vi "Sift Flush Loop.vi"(8 "error in (no error)":errorcluster, 10 "Stop Notifier":refnum<notifier>, 11 "Sift Client In":refnum<class "Sift Client.lvclass">) -> (0 "error out":errorcluster)   [LabVIEW 2024, in "Sift Stream.lvlib" / "Sift Stream.lvclass"]
uses:
  Sift Stream.lvclass
  <vilib>/Sift/Sift/Sift API/Sift Client.lvclass
  Sift Stream.lvclass/Sift Stream.ctl
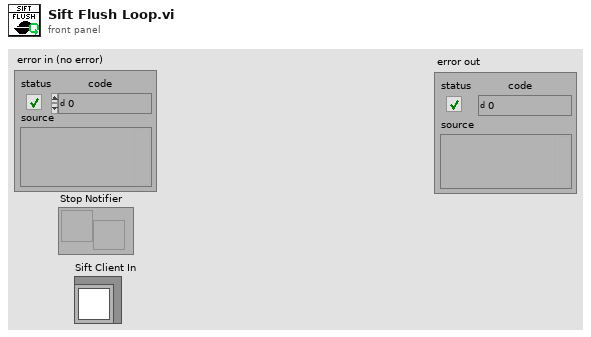
[diagram p1: front panel]
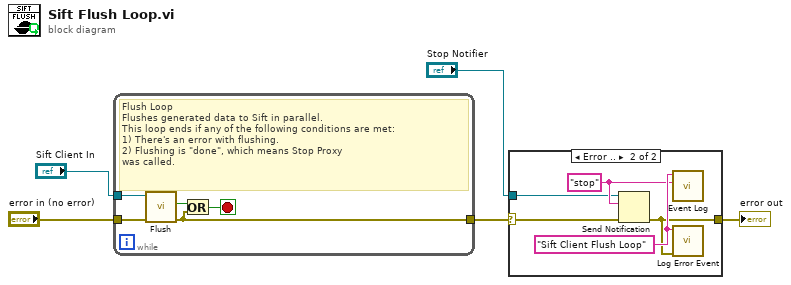
[diagram p0: block diagram]
diagram:
  n1 = while {
    tunnel: [w8] -> w2
    tunnel: "Sift Client In" -> [w7]
    tunnel: "error in (no error)" -> [w6]
    stop <- w10 stop-if-true
    # "Flush Loop\nFlushes generated data to Sift in parallel.\nThis loop ends if any of the following conditions are met:\n1) There's an error with flushing.\n2) Flushing is \"done\", which means Stop Proxy \nwas called."
    n2 = call-dynamic "Flush.vi"("error in (no error)"=w6, "Sift Client in"=w7) -> ("error out"=w8:errorcluster, "Done"=w9:bool)  [unwired: 7 in, 1 out]
    n3 = Or(x=w9, y=w8) -> (x .or. y?=w10:bool)
  }
  n4 = case shown="Error .." w2 {
    selector: w2 -> [w11 w12]
    tunnel: "Stop Notifier" -> [_ w14]
    tunnel: [w11 w13] -> w1
    frame No Error {
    }
    frame Error {
      w16 = "Sift Client Flush Loop"
      w15 = "stop"
      n5 = Send Notification(notification=w15, notifier=w14, error in (no error)=w12) -> (error out=w13:errorcluster)  [unwired: 1 out]
      n6 = call "Event Log.vi"("Event Type"=w15, "Location"=w16) -> ()  [unwired: 10 in]
      n7 = call "Log Error Event.vi"("error in (no error)"=w13, "Location"=w16) -> ()  [unwired: 10 in]
    }
  }
  "error out" <- w1
